vi "Teleop.vi"(10 "Match Info":T1={"Autonomous Elapsed Seconds"=0.0, "TeleOp Elapsed Seconds"=0.0, "Disabled Elapsed Seconds"=0.0, "Visited Autonomous"=FALSE, "Visited TeleOp"=FALSE, "Visited Disabled"=FALSE, "Autonomous Settings"={"Autonomous Style"=enum."Independent", "VI Refnum"=refnum}}, 11 "Call Context":T2) -> ()   [LabVIEW 2015]
doc: "This VI is called for each TeleOp packet received from the DS where the robot is not disabled. It is often used to read from the joysticks and update I/O or to update setpoints for timed control loops. It should complete and return within 20 milliseconds or it may miss DS packets."
uses:
  <vilib>/Rock Robotics/WPI/DriverStation/WPI_DriverStationDerivedRobotMode.ctl
  <vilib>/Rock Robotics/WPI/DriverStation/WPI_DriverStationMatch Info.ctl
  <vilib>/Rock Robotics/WPI/Solenoid/WPI_SolenoidValue.ctl
  <vilib>/Rock Robotics/WPI/Utilities/WPI_GetSetVariantRefNum.vi
  <vilib>/Rock Robotics/Network Tables/NT Read Boolean.vi
  <vilib>/Rock Robotics/Network Tables/NT Read Number.vi
  <vilib>/Rock Robotics/Network Tables/NT Write Numeric Array.vi
  Robot Global Data.vi
  <vilib>/Rock Robotics/WPI/Solenoid/Deprecated/WPI_SolenoidGetBool.vi
  <vilib>/Rock Robotics/WPI/Solenoid/WPI_SolenoidSetEnum.vi
panel:
  out "Sample Slider 0":dbl(slide) scale=0.0..5.0
  out "Sample Boolean 1":bool
  out "Sample Boolean 0":bool
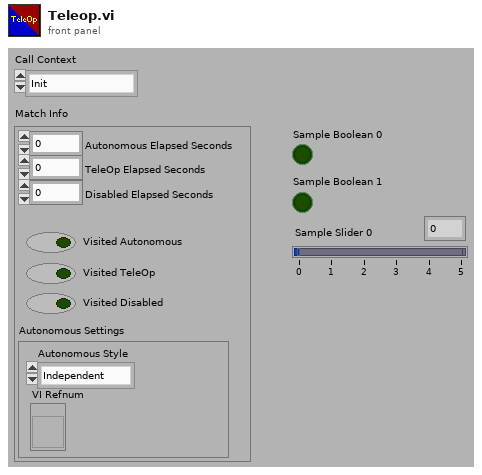
[diagram p1: front panel]
types:
  T1 = typedef "WPI_DriverStationMatch Info.ctl" = cluster{"Autonomous Elapsed Seconds":dbl, "TeleOp Elapsed Seconds":dbl, "Disabled Elapsed Seconds":dbl, "Visited Autonomous":bool, "Visited TeleOp":bool, "Visited Disabled":bool, "Autonomous Settings":cluster{"Autonomous Style":enum16{"Iterative", "Independent"}, "VI Refnum":refnum<vi>}}
  T2 = typedef "WPI_DriverStationDerivedRobotMode.ctl" = enum16{"Init", "Execute", "Stop"}
  T3 = typedef "WPI_JoystickDevRef.ctl" = cluster{"Device":T4}
  T4 = typedef "WPI_JoystickDeviceEnum.ctl" = enum16{"USB 0", "USB 1", "USB 2", "USB 3", "USB 4", "USB 5"}
  T5 = typedef "WPI_MotorControlDeviceRef.ctl" = cluster{"DeviceStatus":errorcluster, "Type":T6, "PWM":cluster{"PWM Channel":T7, "DeadBand":T8}, "CAN":cluster{"Device Number":u8, "Control Mode":T9, "Semaphore":T10, "Max Vout":dbl, "TalonSRX Control Mode":T11}, "Invert":bool}
  T6 = typedef "WPI_MotorControlType.ctl" = enum16{"PWM", "CAN", "CANTalonSRX"}
  T7 = typedef "FPGA_DIOPWMChannel.ctl" = enum8{"PWM 0", "PWM 1", "PWM 2", "PWM 3", "PWM 4", "PWM 5", "PWM 6", "PWM 7", "PWM 8", "PWM 9", "PWM MXP 0", "PWM MXP 1", "PWM MXP 2", "PWM MXP 3", "PWM MXP 4", "PWM MXP 5", "PWM MXP 6", "PWM MXP 7", "PWM MXP 8", "PWM MXP 9", "Invalid"}
  T8 = typedef "WPI_PWMDeadband.ctl" = cluster{"Name":string, "maxPositivePwm":i32, "minPositivePwm":i32, "centerPwm":i32, "maxNegativePwm":i32, "minNegativePwm":i32, "angularRange":u16}
  T9 = typedef "WPI_CANJaguar_ControlMode.ctl" = enum8{"Percent VBus", "Current", "Speed", "Position", "Voltage"}
  T10 = typedef "Semaphore RefNum" = refnum<k1>
  T11 = typedef "WPI_CANTalonSRX_APIControlMode.ctl" = enum8{"Percent VBus", "Speed", "Position", "Slave", "Unchanged / Invalid", "Voltage Compensation", "Current", "Motion Profile"}
  T12 = typedef "WPI_RobotDriveDevRef.ctl" = cluster{"DevStatus":errorcluster, "Motors[]":T5[], "Square Inputs":bool, "Max Output":dbl}
  T13 = typedef "WPI_SolenoidDevRef.ctl" = cluster{"DevStatus":errorcluster, "Pneumatics Control Module":u8, "Forward Solenoid Channel":T14, "Reverse Solenoid Channel":T14}
  T14 = typedef "WPI_SolenoidChannel.ctl" = enum8{"Solenoid 0", "Solenoid 1", "Solenoid 2", "Solenoid 3", "Solenoid 4", "Solenoid 5", "Solenoid 6", "Solenoid 7", "Invalid"}
  T15 = typedef "WPI_SolenoidValue.ctl" = enum16{"Off", "On", "Forward", "Reverse"}
  T16 = typedef "WPI_DigitalInputDevRef.ctl" = cluster{"DevStatus":errorcluster, "DIO Channel":T17}
  T17 = typedef "FPGA_DIOChannel.ctl" = enum8{"DIO 0", "DIO 1", "DIO 2", "DIO 3", "DIO 4", "DIO 5", "DIO 6", "DIO 7", "DIO 8", "DIO 9", "DIO MXP 0", "DIO MXP 1", "DIO MXP 2", "DIO MXP 3", "DIO MXP 4", "DIO MXP 5", "DIO MXP 6", "DIO MXP 7", "DIO MXP 8", "DIO MXP 9", "DIO MXP 10", "DIO MXP 11", "DIO MXP 12", "DIO MXP 13", "DIO MXP 14", "DIO MXP 15", "Invalid"}
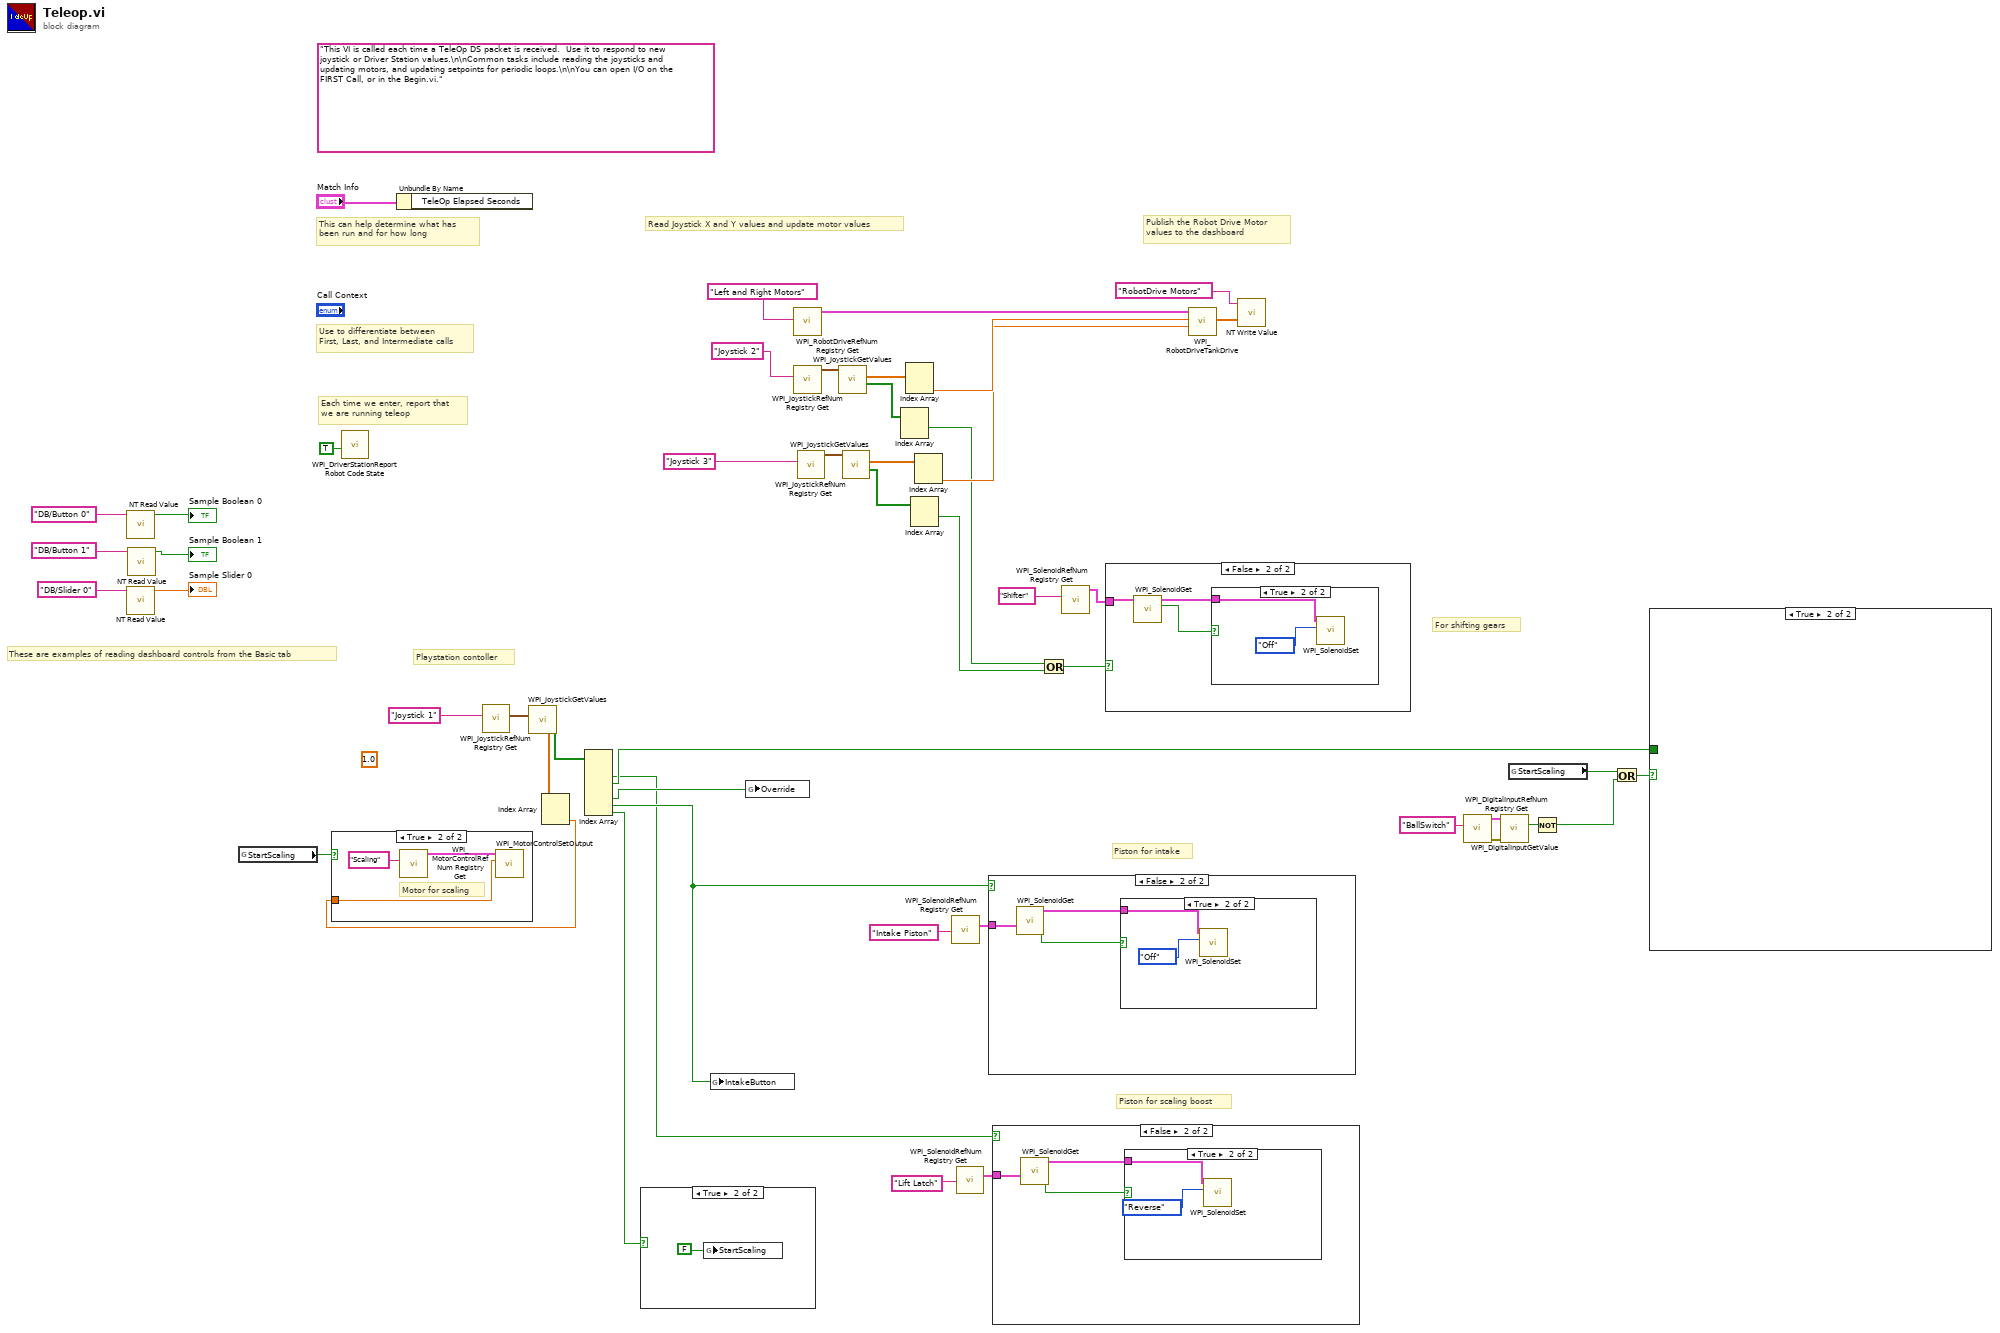
[diagram p0: block diagram]
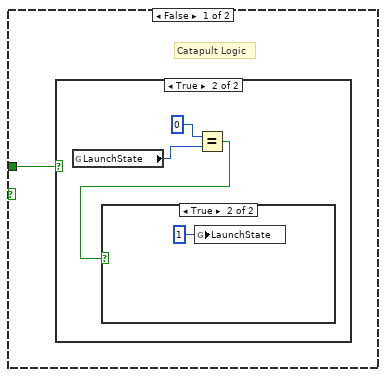
[diagram p3: hidden frame]
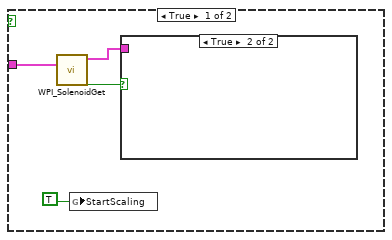
[diagram p7: hidden frame]
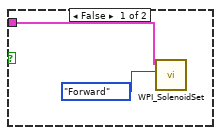
[diagram p8: hidden frame]
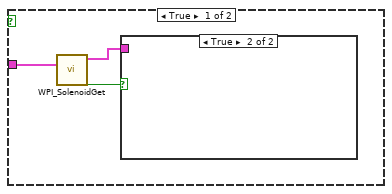
[diagram p10: hidden frame]
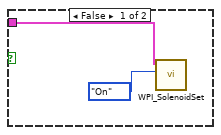
[diagram p11: hidden frame]
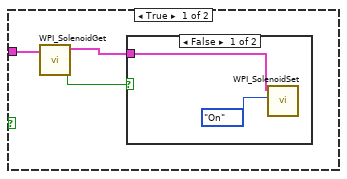
[diagram p13: hidden frame]
diagram:
  (unwired) 1.0 ("Motor Output")
  (unwired) "This VI is called each time a TeleOp DS packet is received.  Use it to respond to new joystick or Driver Station values.\n\nCommon tasks include reading the joysticks and updating motors, and updating setpoints for periodic loops.\n\nYou can open I/O on the FIRST Call, or in the Begin.vi."
  # "Piston for scaling boost"
  # "Piston for intake"
  # "For shifting gears"
  # "Playstation contoller"
  # "These are examples of reading dashboard controls from the Basic tab"
  # "Publish the Robot Drive Motor\nvalues to the dashboard"
  # "Each time we enter, report that\nwe are running teleop"
  # "Use to differentiate between\nFirst, Last, and Intermediate calls"
  # "This can help determine what has\nbeen run and for how long"
  # "Read Joystick X and Y values and update motor values"
  n1 = call-poly <vilib>:"NT Read Value.vi"("Name"="DB/Button 0" ("refnum name")) -> ("Boolean"=→"Sample Boolean 0":bool)  [unwired: 9 in, 1 out]
  n2 = call-poly <vilib>:"NT Read Value.vi"("Name"="DB/Slider 0" ("refnum name")) -> ("Numeric"=→"Sample Slider 0":dbl)  [unwired: 9 in, 1 out]
  n3 = call-poly <vilib>:"NT Read Value.vi"("Name"="DB/Button 1" ("refnum name")) -> ("Boolean"=→"Sample Boolean 1":bool)  [unwired: 9 in, 1 out]
  n4 = global read "Robot Global Data.vi" "StartScaling"() -> (w1:bool)
  n5 = call <vilib>:"WPI_DriverStationReport Robot Code State.vi"("TeleOp"=TRUE ("Autonomous")) -> ()  [unwired: 10 in, 1 out]
  n6 = Unbundle By Name("Match Info") -> ()  [unwired: 1 out]
  n7 = call <vilib>:"WPI_JoystickRefNum Registry Get.vi"("refnum name"="Joystick 1") -> ("JoystickDevRef"=w31:T3)  [unwired: 1 in, 9 out]
  n8 = call <vilib>:"WPI_JoystickGetValues.vi"("JoystickDevRef"=w31) -> ("Buttons"=w29:bool[], "Axes"=w30:dbl[])  [unwired: 6 in, 3 out]
  n9 = Index Array(array=w30) -> (element #2=w2:dbl)  [unwired: 2 in, 1 out]
  n10 = case shown="True" w1 {
    tunnel: w2 -> [_ w50]
    frame False {
    }
    frame True {
      # "Motor for scaling"
      n11 = call <vilib>:"WPI_MotorControlRefNum Registry Get.vi"("refnum name"="Scaling") -> ("MotorControlDevRef"=w52:T5)  [unwired: 9 in, 1 out]
      n12 = call <vilib>:"WPI_MotorControlSetOutput.vi"("Output"=w50, "MotorControlDevRef"=w52) -> ()  [unwired: 7 in, 3 out]
    }
  }
  n13 = Index Array(array=w29) -> (element #2=w11:bool, element #3=w15:bool, element #5=w14:bool, element #6=w16:bool, element #7=w10:bool)  [unwired: 7 in, 2 out]
  n14 = case shown="True" w10 {
    frame False {
    }
    frame True {
      n15 = global write "Robot Global Data.vi" "StartScaling"(FALSE ("Override")) -> ()
    }
  }
  n16 = global write "Robot Global Data.vi" "IntakeButton"(w16) -> ()
  n17 = global write "Robot Global Data.vi" "Override"(w14) -> ()
  n18 = call <vilib>:"WPI_RobotDriveRefNum Registry Get.vi"("refnum name"="Left and Right Motors") -> ("RobotDriveDevRef"=w47:T12)  [unwired: 1 in, 9 out]
  n19 = call <vilib>:"WPI_JoystickRefNum Registry Get.vi"("refnum name"="Joystick 2") -> ("JoystickDevRef"=w45:T3)  [unwired: 1 in, 9 out]
  n20 = call <vilib>:"WPI_JoystickRefNum Registry Get.vi"("refnum name"="Joystick 3") -> ("JoystickDevRef"=w34:T3)  [unwired: 1 in, 9 out]
  n21 = call <vilib>:"WPI_JoystickGetValues.vi"("JoystickDevRef"=w45) -> ("Buttons"=w25:bool[], "Axes"=w43:dbl[])  [unwired: 6 in, 3 out]
  n22 = call <vilib>:"WPI_JoystickGetValues.vi"("JoystickDevRef"=w34) -> ("Buttons"=w24:bool[], "Axes"=w33:dbl[])  [unwired: 6 in, 3 out]
  n23 = Index Array(array=w25) -> (element #1=w20:bool)  [unwired: 2 in, 1 out]
  n24 = Index Array(array=w43) -> (element #2=w27:dbl)  [unwired: 2 in, 1 out]
  n25 = Index Array(array=w24) -> (element #1=w19:bool)  [unwired: 2 in, 1 out]
  n26 = Index Array(array=w33) -> (element #2=w26:dbl)  [unwired: 2 in, 1 out]
  n27 = call <vilib>:"WPI_SolenoidRefNum Registry Get.vi"("refnum name"="Intake Piston") -> ("SolenoidDevRef"=w17:T13)  [unwired: 9 in, 1 out]
  n28 = call <vilib>:"WPI_SolenoidRefNum Registry Get.vi"("refnum name"="Lift Latch") -> ("SolenoidDevRef"=w12:T13)  [unwired: 9 in, 1 out]
  n29 = case shown="False" w16 {
    tunnel: w17 -> [w56 w61]
    frame True {
      n30 = call-poly <vilib>:"WPI_SolenoidGet.vi"("SolenoidDevRef"=w56) -> ("Value"=w54:bool, "SolenoidDevRef"=w55:T13)  [unwired: 8 in, 1 out]
      n31 = case shown="True" w54 {
        tunnel: w55 -> [w57 _]
        frame False {
          n32 = call-poly <vilib>:"WPI_SolenoidSet.vi"("Value"=WPI_SolenoidValue."On", "SolenoidDevRef"=w57) -> ()  [unwired: 8 in, 2 out]
        }
        frame True {
        }
      }
    }
    frame False {
      n33 = call-poly <vilib>:"WPI_SolenoidGet.vi"("SolenoidDevRef"=w61) -> ("Value"=w59:bool, "SolenoidDevRef"=w60:T13)  [unwired: 8 in, 1 out]
      n34 = case shown="True" w59 {
        tunnel: w60 -> [_ w63]
        frame False {
        }
        frame True {
          n35 = call-poly <vilib>:"WPI_SolenoidSet.vi"("Value"=WPI_SolenoidValue."Off", "SolenoidDevRef"=w63) -> ()  [unwired: 8 in, 2 out]
        }
      }
    }
  }
  n36 = case shown="False" w11 {
    tunnel: w12 -> [w67 w72]
    frame True {
      n37 = call-poly <vilib>:"WPI_SolenoidGet.vi"("SolenoidDevRef"=w67) -> ("Value"=w65:bool, "SolenoidDevRef"=w66:T13)  [unwired: 8 in, 1 out]
      n38 = global write "Robot Global Data.vi" "StartScaling"(TRUE ("Override")) -> ()
      n39 = case shown="True" w65 {
        tunnel: w66 -> [w68 _]
        frame False {
          n40 = call-poly <vilib>:"WPI_SolenoidSet.vi"("Value"=WPI_SolenoidValue."Forward", "SolenoidDevRef"=w68) -> ()  [unwired: 8 in, 2 out]
        }
        frame True {
        }
      }
    }
    frame False {
      n41 = call-poly <vilib>:"WPI_SolenoidGet.vi"("SolenoidDevRef"=w72) -> ("Value"=w70:bool, "SolenoidDevRef"=w71:T13)  [unwired: 8 in, 1 out]
      n42 = case shown="True" w70 {
        tunnel: w71 -> [_ w74]
        frame False {
        }
        frame True {
          n43 = call-poly <vilib>:"WPI_SolenoidSet.vi"("Value"=WPI_SolenoidValue."Reverse", "SolenoidDevRef"=w74) -> ()  [unwired: 8 in, 2 out]
        }
      }
    }
  }
  n44 = Or(x=w20, y=w19) -> (x .or. y?=w21:bool)
  n45 = call <vilib>:"WPI_SolenoidRefNum Registry Get.vi"("refnum name"="Shifter") -> ("SolenoidDevRef"=w23:T13)  [unwired: 9 in, 1 out]
  n46 = case shown="False" w21 {
    tunnel: w23 -> [w75 w80]
    frame True {
      n47 = call-poly <vilib>:"WPI_SolenoidGet.vi"("SolenoidDevRef"=w75) -> ("Value"=w76:bool, "SolenoidDevRef"=w77:T13)  [unwired: 8 in, 1 out]
      n48 = case shown="False" w76 {
        tunnel: w77 -> [w78 _]
        frame False {
          n49 = call-poly <vilib>:"WPI_SolenoidSet.vi"("Value"=WPI_SolenoidValue."On", "SolenoidDevRef"=w78) -> ()  [unwired: 8 in, 2 out]
        }
        frame True {
        }
      }
    }
    frame False {
      n50 = call-poly <vilib>:"WPI_SolenoidGet.vi"("SolenoidDevRef"=w80) -> ("Value"=w81:bool, "SolenoidDevRef"=w82:T13)  [unwired: 8 in, 1 out]
      n51 = case shown="True" w81 {
        tunnel: w82 -> [_ w84]
        frame False {
        }
        frame True {
          n52 = call-poly <vilib>:"WPI_SolenoidSet.vi"("Value"=WPI_SolenoidValue."Off", "SolenoidDevRef"=w84) -> ()  [unwired: 8 in, 2 out]
        }
      }
    }
  }
  n53 = call <vilib>:"WPI_RobotDriveTankDrive.vi"("Right axis value"=w26, "Left axis value"=w27, "RobotDriveDevRef"=w47) -> ("Motor Values"=w36:dbl[])  [unwired: 6 in, 2 out]
  n54 = call-poly <vilib>:"NT Write Value.vi"("Numeric Array"=w36, "Name"="RobotDrive Motors") -> ()  [unwired: 9 in, 1 out]
  n55 = call <vilib>:"WPI_DigitalInputRefNum Registry Get.vi"("refnum name"="BallSwitch") -> ("error out"=w7:errorcluster, "DigitalInputDevRef"=w6:T16)  [unwired: 9 in]
  n56 = call <vilib>:"WPI_DigitalInputGetValue.vi"("error in (no error)"=w7, "DigitalInputDevRef"=w6) -> ("Value"=w5:bool)  [unwired: 7 in, 2 out]
  n57 = global read "Robot Global Data.vi" "StartScaling"() -> (w8:bool)
  n58 = Not(x=w5) -> (.not. x?=w4:bool)
  n59 = Or(x=w8, y=w4) -> (x .or. y?=w9:bool)
  n60 = case shown="True" w9 {
    tunnel: w15 -> [w85 _]
    frame False {
      # "Catapult Logic"
      n61 = case shown="True" w85 {
        frame False {
        }
        frame True {
          n62 = global read "Robot Global Data.vi" "LaunchState"() -> (w87:u8)
          n63 = Equal?(x=u8 0, y=w87) -> (x = y?=w86:bool)
          n64 = case shown="True" w86 {
            frame False {
            }
            frame True {
              n65 = global write "Robot Global Data.vi" "LaunchState"(u8 1 ("LaunchState")) -> ()
            }
          }
        }
      }
    }
    frame True {
    }
  }
